vi "CtrlTreeOpenUptoSelectedItems.vi"(8 "error in (no error)":errorcluster, 11 "TreeControl in":refnum<vi>) -> (0 "error out":errorcluster, 3 "TreeControl out":refnum<vi>)   [LabVIEW 2019]
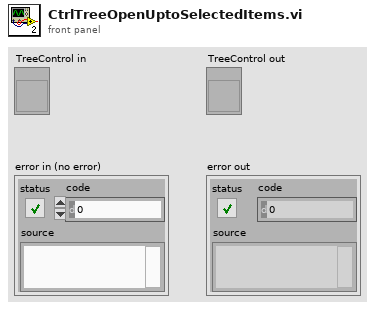
[diagram p1: front panel]
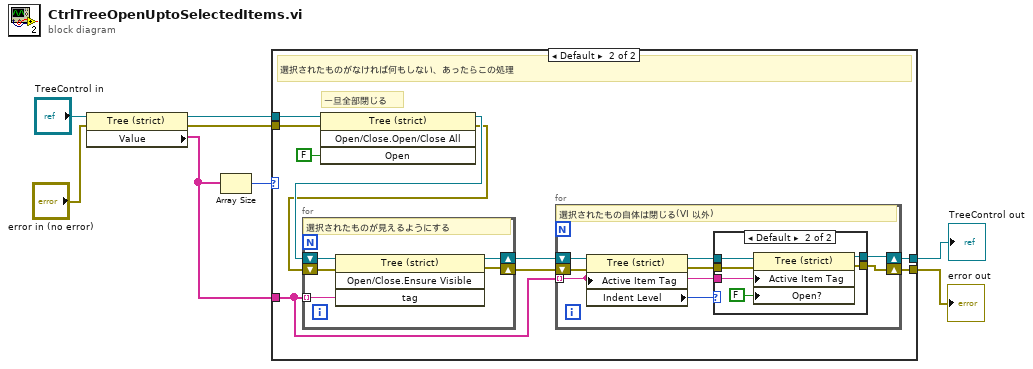
[diagram p0: block diagram]
diagram:
  n1 = property class="Tree (strict)"(reference="TreeControl in", error in="error in (no error)") -> (reference out=w6:refnum<vi>, error out=w3:errorcluster, "Value"=w5:string[])
  n2 = Array Size(array=w5) -> (size(s)=w7:i32)
  n3 = case shown="Default" w7 {
    tunnel: w6 -> [w10 w20]
    tunnel: w5 -> [_ w16]
    tunnel: w3 -> [w9 w15]
    tunnel: [w9 w12] -> w2
    tunnel: [w10 w11] -> w1
    frame 0 {
    }
    frame Default {
      # "一旦全部閉じる"
      # "選択されたものがなければ何もしない、あったらこの処理"
      n4 = invoke class="Tree (strict)" method="Open/Close.Open/Close All"(reference=w20, error in=w15, "Open"=FALSE ("Open?")) -> (reference out=w18:refnum<vi>, error out=w14:errorcluster)  [unwired: 1 in, 2 out]
      n5 = for {
        tunnel: w16 -> [w40] mode=indexing
        shift-right: [w39] -> w17
        shift-left: w18 -> [w41]
        shift-right: [w37] -> w13
        shift-left: w14 -> [w38]
        # "選択されたものが見えるようにする"
        n6 = invoke class="Tree (strict)" method="Open/Close.Ensure Visible"(reference=w41, error in=w38, "tag"=w40) -> (reference out=w39:refnum<vi>, error out=w37:errorcluster)  [unwired: 1 in, 2 out]
      }
      n7 = for {
        shift-right: [w27] -> w11
        shift-left: w17 -> [w28]
        tunnel: w16 -> [w25] mode=indexing
        shift-right: [w21] -> w12
        shift-left: w13 -> [w23]
        # "選択されたもの自体は閉じる(VI 以外)"
        n8 = property class="Tree (strict)"(reference=w28, error in=w23, "Active Item Tag"=w25) -> (reference out=w26:refnum<vi>, error out=w22:errorcluster, "Indent Level"=w24:i32)
        n9 = case shown="Default" w24 {
          tunnel: [w30 w36] -> w27
          tunnel: w26 -> [w30 w34]
          tunnel: w25 -> [_ w33]
          tunnel: w22 -> [w29 w32]
          tunnel: [w29 w31] -> w21
          frame 1 {
          }
          frame Default {
            n10 = property class="Tree (strict)"(reference=w34, error in=w32, "Active Item Tag"=w33, "Open?"=FALSE ("Active Item:Open?")) -> (reference out=w36:refnum<vi>, error out=w31:errorcluster)
          }
        }
      }
    }
  }
  "error out" <- w2
  "TreeControl out" <- w1
